vi "DAC set current.vi"(8 "Ranging byte":u8, 10 "DAC output (µA)":dbl) -> (0 "Voltage out":dbl)   [LabVIEW 2013]
panel:
  in  "Galv. cal. data":dbl[][](array[numeric])
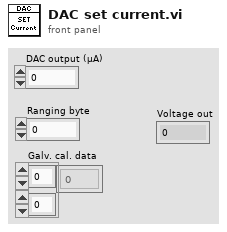
[diagram p1: front panel]
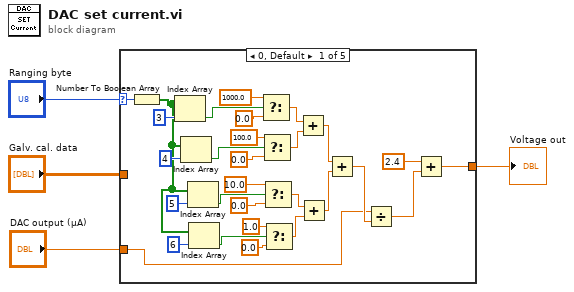
[diagram p0: block diagram]
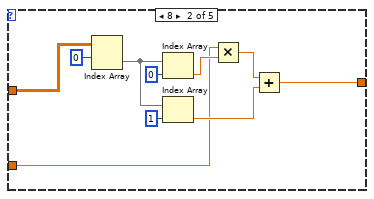
[diagram p2: hidden frame]
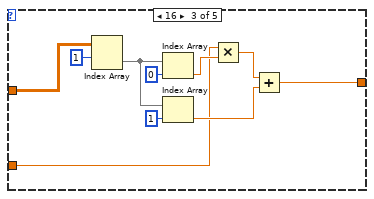
[diagram p3: hidden frame]
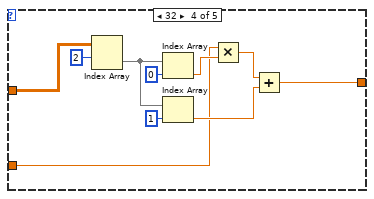
[diagram p4: hidden frame]
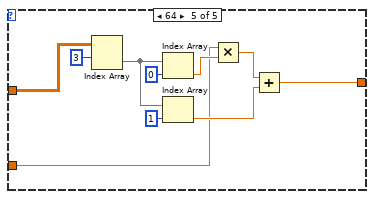
[diagram p5: hidden frame]
diagram:
  n1 = case shown="0, Default" "Ranging byte" {
    selector: "Ranging byte" -> [w9 _ _ _ _]
    tunnel: "Galv. cal. data" -> [_ w43 w53 w63 w73]
    tunnel: "DAC output (µA)" -> [w8 w35 w45 w55 w65]
    tunnel: [w7 w34 w44 w54 w64] -> w1
    frame 0, Default {
      n2 = Number To Boolean Array(number=w9) -> (Boolean array=w10:bool[])
      n3 = Index Array(array=w10, index=3) -> (element=w23:bool)
      n4 = Index Array(array=w10, index=4) -> (element=w24:bool)
      n5 = Index Array(array=w10, index=5) -> (element=w25:bool)
      n6 = Index Array(array=w10, index=6) -> (element=w26:bool)
      n7 = Select(t=1000.0, s=w23, f=0.0) -> (s? t:f=w27:dbl)
      n8 = Select(t=100.0, s=w24, f=0.0) -> (s? t:f=w28:dbl)
      n9 = Select(t=10.0, s=w25, f=0.0) -> (s? t:f=w29:dbl)
      n10 = Select(t=1.0, s=w26, f=0.0) -> (s? t:f=w30:dbl)
      n11 = Add(x=w27, y=w28) -> (x+y=w31:dbl)
      n12 = Add(x=w29, y=w30) -> (x+y=w32:dbl)
      n13 = Add(x=w31, y=w32) -> (x+y=w33:dbl)
      n14 = Divide(x=w8, y=w33) -> (x/y=w5:dbl)
      n15 = Add(x=2.4 ("y"), y=w5) -> (x+y=w7:dbl)
    }
    frame 8 {
      n16 = Index Array(array=w43, index (row)=0 ("index")) -> (element=w39:dbl[])  [unwired: 1 in]
      n17 = Index Array(array=w39, index=0) -> (element=w38:dbl)
      n18 = Index Array(array=w39, index=1) -> (element=w37:dbl)
      n19 = Multiply(x=w35, y=w38) -> (x*y=w36:dbl)
      n20 = Add(x=w36, y=w37) -> (x+y=w34:dbl)
    }
    frame 16 {
      n21 = Index Array(array=w53, index (row)=1 ("index")) -> (element=w49:dbl[])  [unwired: 1 in]
      n22 = Index Array(array=w49, index=0) -> (element=w48:dbl)
      n23 = Index Array(array=w49, index=1) -> (element=w47:dbl)
      n24 = Multiply(x=w45, y=w48) -> (x*y=w46:dbl)
      n25 = Add(x=w46, y=w47) -> (x+y=w44:dbl)
    }
    frame 32 {
      n26 = Index Array(array=w63, index (row)=2 ("index")) -> (element=w59:dbl[])  [unwired: 1 in]
      n27 = Index Array(array=w59, index=0) -> (element=w58:dbl)
      n28 = Index Array(array=w59, index=1) -> (element=w57:dbl)
      n29 = Multiply(x=w55, y=w58) -> (x*y=w56:dbl)
      n30 = Add(x=w56, y=w57) -> (x+y=w54:dbl)
    }
    frame 64 {
      n31 = Index Array(array=w73, index (row)=3 ("index")) -> (element=w69:dbl[])  [unwired: 1 in]
      n32 = Index Array(array=w69, index=0) -> (element=w68:dbl)
      n33 = Index Array(array=w69, index=1) -> (element=w67:dbl)
      n34 = Multiply(x=w65, y=w68) -> (x*y=w66:dbl)
      n35 = Add(x=w66, y=w67) -> (x+y=w64:dbl)
    }
  }
  "Voltage out" <- w1
